vi "niDTS GNSS RF Test Initiate.vi"(0 "Template Tx Test Handle in":T1, 11 "error in (no error)":errorcluster) -> (4 "Template Tx Test Handle out":T1, 15 "error out":errorcluster)   [LabVIEW 2014, in "niDTS GNSS.lvlib"]
uses:
  niDTS GNSS.lvlib
  Includes/niDTS GNSS RF Test INC Handle.ctl
  Objects/BASE_class/niDTS GNSS RF Test.lvclass
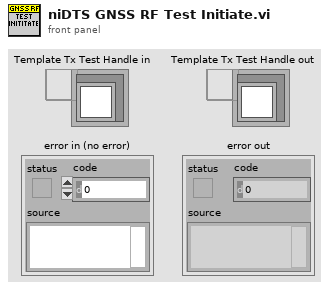
[diagram p1: front panel]
types:
  T1 = typedef "niDTS GNSS.lvlib/niDTS GNSS RF Test INC Handle.ctl" = refnum<data-value>
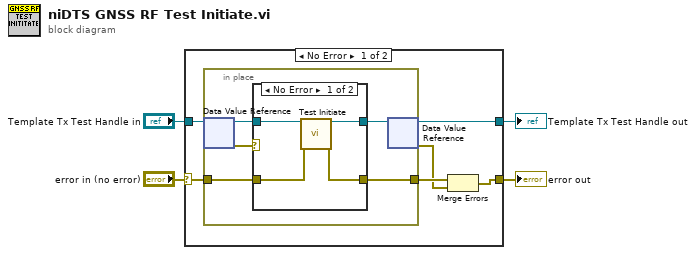
[diagram p0: block diagram]
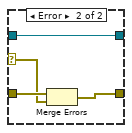
[diagram p2: hidden frame]
diagram:
  n1 = case shown="No Error" "error in (no error)" {
    selector: "error in (no error)" -> [w8 w25]
    tunnel: "Template Tx Test Handle in" -> [w10 w24]
    tunnel: [w9 w24] -> w3
    tunnel: [w7 w25] -> w2
    frame No Error {
      n2 = in-place {
        in-place-border: w8 -> [w12]
        in-place-border: [w11] -> w6
        n3 = in-place-dvr #1(w10) -> (w14:refnum<class "niDTS GNSS RF Test.lvclass">, w15:errorcluster)
        n4 = case shown="No Error" w15 {
          selector: w15 -> [_ w21]
          tunnel: w14 -> [w19 w23]
          tunnel: [w18 w23] -> w13
          tunnel: w12 -> [w17 w22]
          tunnel: [w16 w20] -> w11
          frame No Error {
            n5 = call-dynamic "Test Initiate.vi"("Template Tx Test in"=w19, "error in (no error)"=w17) -> ("Template Tx Test out"=w18:refnum<class "niDTS GNSS RF Test.lvclass">, "error out"=w16:errorcluster)  [unwired: 12 in]
          }
          frame Error {
            n6 = Merge Errors(w22, w21) -> (w20:errorcluster)
          }
        }
        n7 = in-place-dvr #1(w13) -> (w9:T1, w5:errorcluster)
      }
      n8 = Merge Errors(w6, w5) -> (w7:errorcluster)
    }
    frame Error {
    }
  }
  "Template Tx Test Handle out" <- w3
  "error out" <- w2
